vi "niDDC Initiate Acquisition.vi"(8 "error in (no error)":errorcluster, 11 "Class in":refnum<class "7976R_v1.lvclass">) -> (0 "error out":errorcluster, 3 "Class out":refnum<class "7976R_v1.lvclass">)   [LabVIEW 2015, in "7976R_v1.lvclass"]
uses:
  <userlib>/SE-APP-Receiver/NI5772/7976R_v1/7976R_v1.lvclass
  <userlib>/SE-APP-Receiver/NI5772/7976R_v1/7976R_v1.lvclass/7976R_v1.ctl
  <vilib>/Utility/error.llb/Error Cluster From Error Code.vi
  <vilib>/rvi/errors/niLvFpgaAdjustHostInterfaceError.vi
  <vilib>/rvi/interface/nirviReadWriteControl/nirviReadWriteControl.xnode
  <userlib>/SE-APP-Receiver/NI5772/7976R_v1/Private/FPGA VI Reference_DDC_v1.8.ctl
  NiFpgaLv.dll
  <vilib>/rvi/interface/Simulation/niFpgaSimulationCallBeginRW.vi
panel:
  out "DMA Flush Status (0==OK)":u32
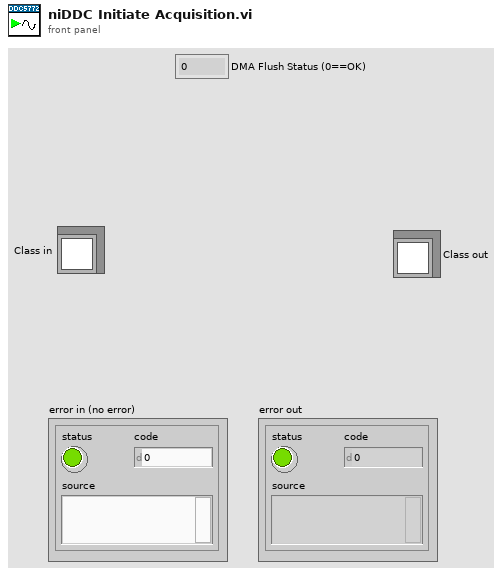
[diagram p1: front panel]
types:
  T1 = typedef "7976R_v1.lvclass/FPGA VI Reference_DDC_v1.8.ctl" = refnum<k20>
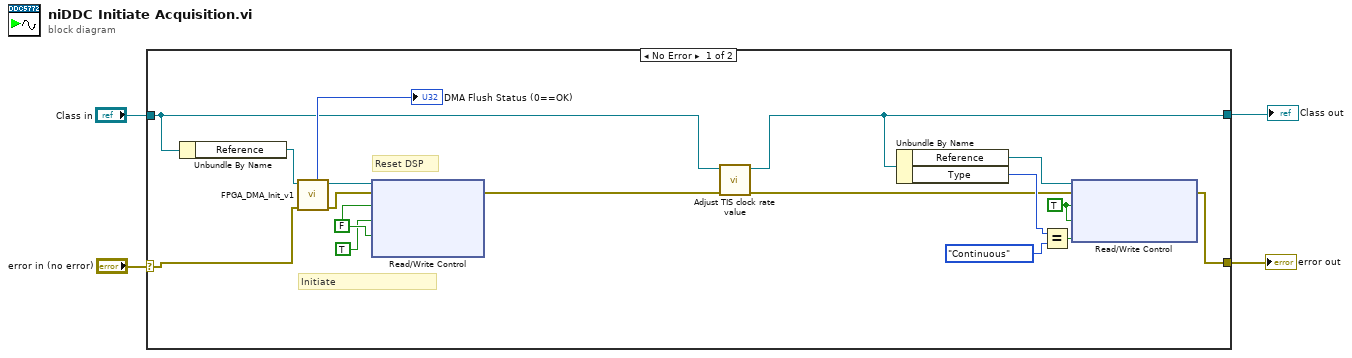
[diagram p0: block diagram]
diagram:
  n1 = case shown="No Error" "error in (no error)" {
    selector: "error in (no error)" -> [w15 w23]
    tunnel: [w11 w23] -> w4
    tunnel: "Class in" -> [w10 w22]
    tunnel: [w7 w22] -> w1
    frame No Error {
      w14 = TRUE ("dbg.stream.enable.1")
      w18 = FALSE
      # "Reset DSP"
      # "Initiate"
      n2 = Unbundle By Name(w10) -> ("Reference"=w16:T1)
      n3 = call <userlib>:"FPGA_DMA_Init_v1.vi"("error in (no error)"=w15, "Refnum in"=w16) -> ("error out"=w19:errorcluster, "Refnum out"=w20:T1, "Remaining"=→"DMA Flush Status (0==OK)":u32)  [unwired: 7 in]
      n4 = xnode "Read/Write Control"("FPGA VI Reference In"=w20, "error in"=w19, "acq.reset"=w18, "acq.reset"=TRUE, "acq.reset"=w18) -> ("error out"=w6:errorcluster)  [unwired: 1 in, 1 out]
      n5 = call <userlib>:"Adjust TIS clock rate value.vi"("error in (no error)"=w6, "7976R_v1 in"=w10) -> ("error out"=w5:errorcluster, "7976R_v1 out"=w7:refnum<class "7976R_v1.lvclass">)  [unwired: 8 in]
      n6 = Unbundle By Name(w7) -> ("Reference"=w9:T1, "Type"=w8:enum16{"Continuous", "Finite"})
      n7 = Equal?(x=w8, y=enum16{"Continuous", "Finite"}."Continuous" ("Acquisition.Type")) -> (x = y?=w12:bool)
      n8 = xnode "Read/Write Control"("FPGA VI Reference In"=w9, "error in"=w5, "dbg.stream.enable.1"=w14, "dbg.stream.enable.2"=w14, "mode.continuous"=w12) -> ("error out"=w11:errorcluster)  [unwired: 1 out]
    }
    frame Error {
    }
  }
  "error out" <- w4
  "Class out" <- w1
